vi "Actor Core.vi"(8 "error in":errorcluster, 11 "Red Pitaya in":refnum<class "Red Pitaya.lvclass">) -> (0 "error out":errorcluster, 3 "Actor out":refnum<class "Actor.lvclass">)   [LabVIEW 2015, in "Red Pitaya.lvclass"]
doc: "(<B>Filename</B>: Actor Framework.lvlib:Actor.lvclass:Actor Core.vi)\n\nReceives messages to the actor, reacts to them, and initiates any error handling that may shut the actor down.\n\nDescendant classes may override this VI to append parallel tasks for the actor to complete while it handles messages. Overrides use the Call Parent Method node."
uses:
  Red Pitaya.lvclass
  <vilib>/ActorFramework/Actor/Actor.lvclass
  Red Pitaya.lvclass/Red Pitaya.ctl
  Mag Lab Measure/Mag Lab Root/Mag Lab Root.lvclass/Mag Lab Root.ctl
  <vilib>/ActorFramework/Actor/Actor.lvclass/Actor.ctl
  <vilib>/ActorFramework/Message Enqueuer/Message Enqueuer.lvclass/Message Enqueuer.ctl
  Mag Lab Measure/Hardware/Mag Lab Digitizer Messages/Arm Msg/Arm Msg.lvclass/Arm Msg.ctl
  <vilib>/ActorFramework/Message Enqueuer/Init from Existing Queue.vi
  <vilib>/ActorFramework/Message Enqueuer/Enqueue.vi
  <vilib>/ActorFramework/Message Priority Queue/Priority Enqueue.vi
  Mag Lab Measure/Hardware/Digitizer/Mag Lab Digitizer.lvclass
  <vilib>/ActorFramework/Message Enqueuer/Message Enqueuer.lvclass
  Mag Lab Measure/Hardware/Mag Lab Digitizer Messages/Arm Msg/Arm Msg.lvclass
  Mag Lab Measure/Mag Lab Root/Mag Lab Root.lvclass
panel:
  in  "Arm":bool
  out "Trigger state":bool
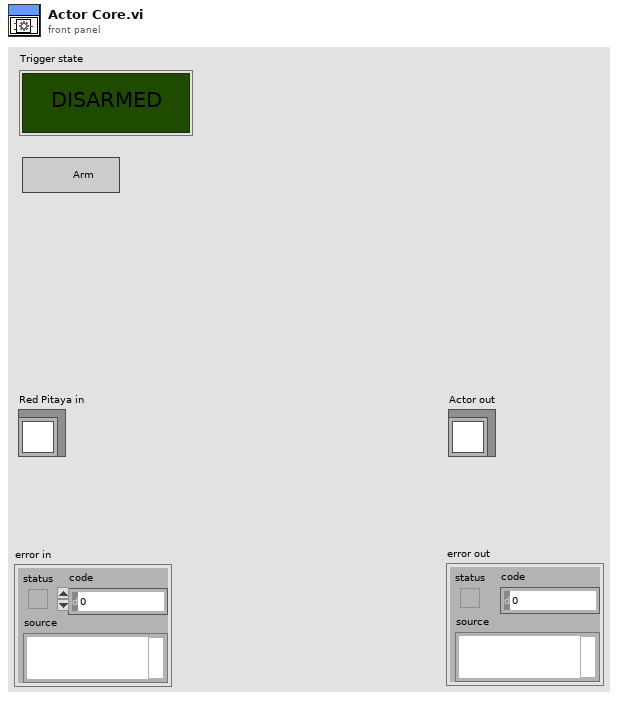
[diagram p1: front panel]
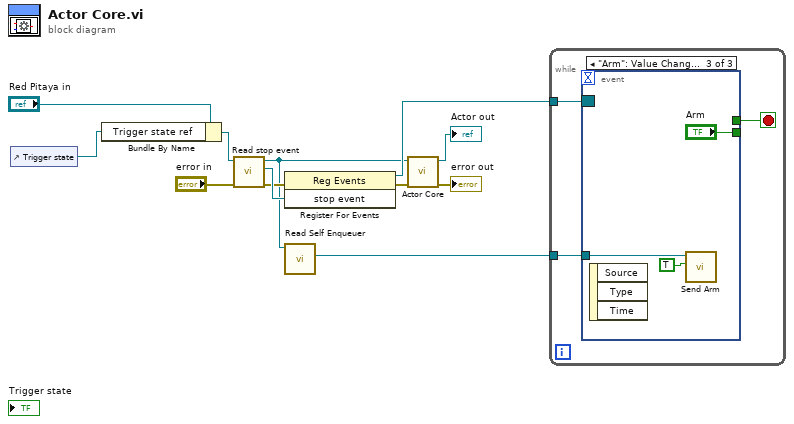
[diagram p0: block diagram]
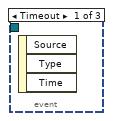
[diagram p2: hidden frame]
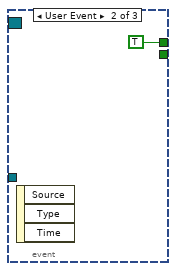
[diagram p3: hidden frame]
diagram:
  n1 = control-ref of="Trigger state"() -> (w3:refnum<vi>)
  n2 = Bundle By Name(cluster="Red Pitaya in", "Trigger state ref"=w3) -> (w4:refnum<class "Red Pitaya.lvclass">)
  n3 = call "Read stop event.vi"("error in (no error)"="error in", "Mag Lab Root in"=w4) -> ("error out"=w7:errorcluster, "stop event"=w9:refnum<user-event>, "Mag Lab Root out"=w2:refnum<class "Red Pitaya.lvclass">)  [unwired: 7 in]
  n4 = register-events(error in=w7, w9) -> (reference out=w5:refnum<event-registration>, error out=w6:errorcluster)  [unwired: 1 in]
  n5 = call <vilib>:"Read Self Enqueuer.vi"("Actor"=w2) -> ("Self Enqueuer"=w1:refnum<class "Message Enqueuer.lvclass">)  [unwired: 10 in]
  n6 = call-parent "Actor Core.vi"("error in"=w6, "Mag Lab Measure Base in"=w2) -> ("error out"=→"error out":errorcluster, "Actor out"=→"Actor out":refnum<class "Actor.lvclass">)  [unwired: 8 in]
  n7 = while {
    tunnel: w5 -> [w15]
    tunnel: w1 -> [w13]
    stop <- w14 stop-if-true
    n8 = event shown="[2] \"Arm\": Value Change" {
      selector: w15 -> [_ _ _]
      dyn-events: _ -> [_ _ _]
      timeout: _ -> [_ _ _]
      tunnel: [_ TRUE _] -> w14
      tunnel: [_ _ "Arm"] -> _
      tunnel: w13 -> [_ _ w18]
      event Timeout {
        n9 = event-data() -> ()  [unwired: 1 in, 3 out]
      }
      event User Event {
        n10 = event-data() -> ()  [unwired: 1 in, 3 out]
      }
      event "Arm": Value Change {
        n11 = event-data() -> ()  [unwired: 1 in, 3 out]
        n12 = call "Send Arm.vi"("Arm"=TRUE, "Message Enqueuer"=w18) -> ()  [unwired: 8 in, 2 out]
      }
    }
  }
